vi "Get Connection Settings.vi"(8 "error in (no error)":errorcluster, 11 "Item Ref in":T2 format="%.0x") -> (0 "error out":errorcluster, 1 "Connection Settings":T3, 2 "ConSelection":T1, 3 "Item Ref out":T2 format="%.0x")   [LabVIEW 2011, in "Chassis TimeSync System Explorer.lvlib"]
uses:
  Chassis TimeSync System Explorer.lvlib
  <vilib>/NI Veristand/Custom Device API/Custom Device Item Ref.ctl
  Shared/Connection Settings.ctl
  Shared/Mode.ctl
  Shared/External Pin.ctl
  Shared/Routes.ctl
  Shared/Route.ctl
  Connection Selection.ctl
  Shared/Constants.vi
  <vilib>/NI Veristand/Custom Device API/Get Item Property (U16).vi
  <vilib>/NI Veristand/Custom Device API/Custom Device API.lvlib
  Shared/Chassis TimeSync Shared.lvlib
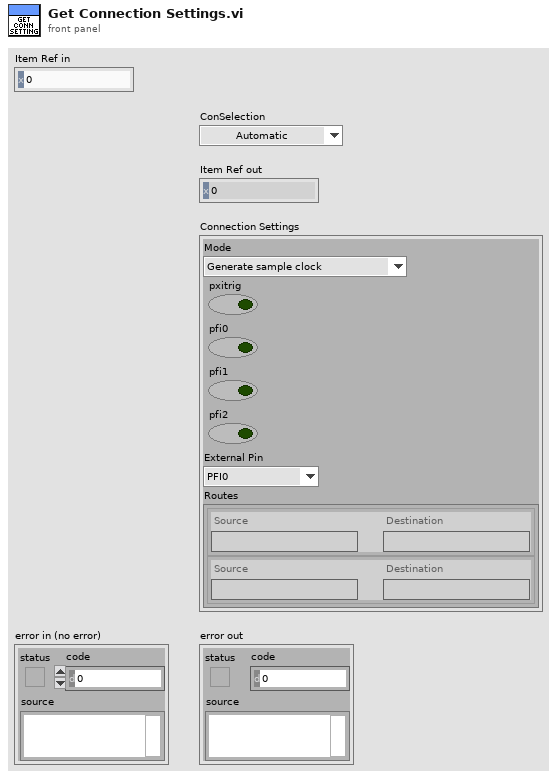
[diagram p1: front panel]
types:
  T1 = typedef "Chassis TimeSync System Explorer.lvlib/Connection Selection.ctl" = enum16{"Automatic", "Custom"}
  T2 = typedef "Custom Device API.lvlib/Custom Device Item Ref.ctl" = u64
  T3 = typedef "Chassis TimeSync Shared.lvlib/Connection Settings.ctl" = cluster{"Mode":T4, "pxitrig":bool, "pfi0":bool, "pfi1":bool, "pfi2":bool, "External Pin":T5, "Routes":T6}
  T4 = typedef "Chassis TimeSync Shared.lvlib/Mode.ctl" = enum16{"Generate sample clock", "Route sample clock out of chassis", "Route sample clock into chassis", "Custom routes"}
  T5 = typedef "Chassis TimeSync Shared.lvlib/External Pin.ctl" = enum16{"PFI0", "PFI1", "PFI2"}
  T6 = typedef "Chassis TimeSync Shared.lvlib/Routes.ctl" = T7[]
  T7 = typedef "Chassis TimeSync Shared.lvlib/Route.ctl" = cluster{"Source":string, "Destination":string}
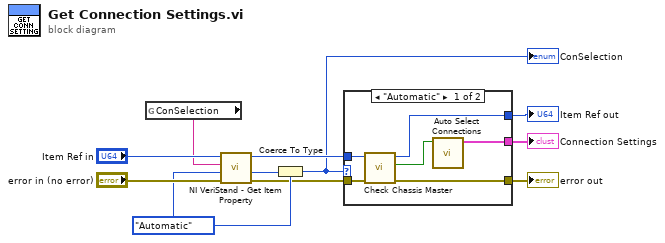
[diagram p0: block diagram]
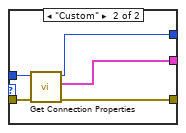
[diagram p2: hidden frame]
diagram:
  w4 = Connection_Selection."Automatic" ("ConSelection")
  n1 = global read "Constants.vi" "ConSelection"() -> (w1:string)
  n2 = call-poly <vilib>:"NI VeriStand - Get Item Property.vi"("error in (no error)"="error in (no error)", "Default Value"=w4, "Property Name"=w1, "Item Ref in"="Item Ref in") -> ("error out"=w2:errorcluster, "Value"=w3:u16, "Item Ref out"=w6:T2)  [unwired: 4 in, 1 out]
  n3 = Coerce To Type(0:w3, 1:w4) -> (2:w5:T1)
  "ConSelection" <- w5
  n4 = case shown="\"Automatic\"" w5 {
    tunnel: w2 -> [w17 w22]
    tunnel: [w13 w21] -> w7
    tunnel: w6 -> [w16 w20]
    tunnel: [w14 w19] -> w8
    tunnel: [w12 w18] -> w10
    frame "Automatic" {
      n5 = call "Check Chassis Master.vi"("error in (no error)"=w17, "Device Item Ref in"=w16) -> ("error out"=w13:errorcluster, "Master?"=w15:bool, "Item Ref out"=w14:T2)  [unwired: 7 in]
      n6 = call "Auto Select Connections.vi"("Master?"=w15) -> ("AutoSelect"=w12:T3)  [unwired: 10 in]
    }
    frame "Custom" {
      n7 = call "Get Connection Properties.vi"("error in (no error)"=w22, "Device Item Ref in"=w20) -> ("error out"=w21:errorcluster, "AutoSelect"=w18:T3, "Item Ref out"=w19:T2)  [unwired: 7 in]
    }
  }
  "Connection Settings" <- w10
  "Item Ref out" <- w8
  "error out" <- w7
